vi "ELVIS III v1.0 RPC Get Session.vi"(8 "error in (no error)":errorcluster) -> (0 "error out":errorcluster, 3 "Session":u32)   [LabVIEW 2021]
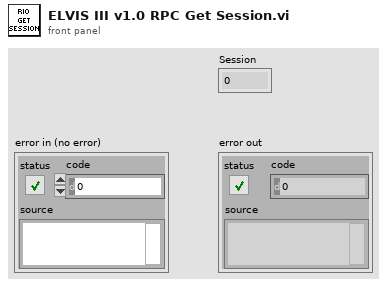
[diagram p1: front panel]
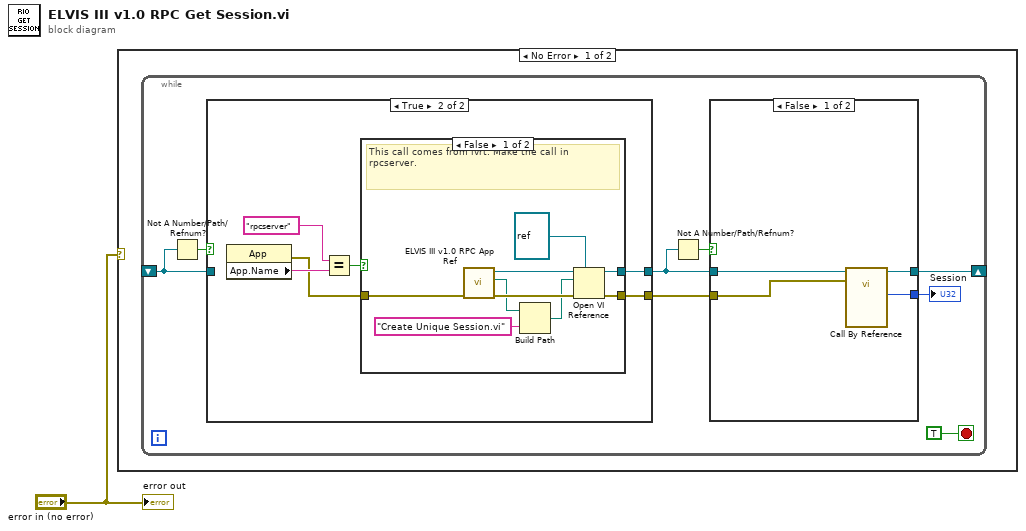
[diagram p0: block diagram]
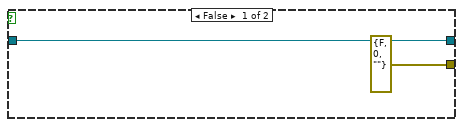
[diagram p2: hidden frame]
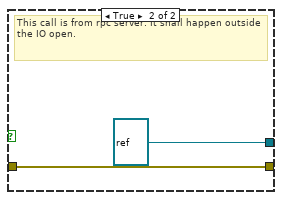
[diagram p3: hidden frame]
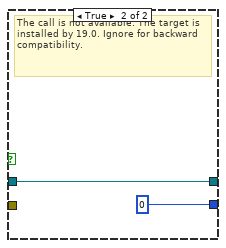
[diagram p4: hidden frame]
diagram:
  n1 = case shown="No Error" "error in (no error)" {
    frame No Error {
      n2 = while {
        shift-right: [w6] -> _
        shift-left: _ -> [w4]
        stop <- TRUE stop-if-true
        n3 = Not A Number/Path/Refnum?(number/path/refnum=w4) -> (NaN/Path/Refnum?=w5:bool)
        n4 = case shown="True" w5 {
          tunnel: [w11 w14] -> w8
          tunnel: w4 -> [w11 _]
          tunnel: [errorcluster {"status"=FALSE, "code"=0, "source"=""} ("error out") w12] -> w3
          frame False {
          }
          frame True {
            n5 = property class="App"() -> (error out=w13:errorcluster, "App.Name"=w17:string)  [unwired: 2 in, 1 out]
            n6 = Equal?(x="rpcserver" ("Application:Name"), y=w17) -> (x = y?=w16:bool)
            n7 = case shown="False" w16 {
              tunnel: [w24 refnum<vi> refnum ("type specifier VI Refnum (for type only)")] -> w14
              tunnel: w13 -> [w22 w27]
              tunnel: [w23 w27] -> w12
              frame False {
                # "This call comes from lvrt. Make the call in rpcserver."
                n8 = call <vilib>:"ELVIS III v1.0 RPC App Ref.vi"() -> ("Lib Path"=w21:path, "RPC Reference"=w19:refnum<vi>)  [unwired: 10 in]
                n9 = Build Path(base path=w21, name or relative path="Create Unique Session.vi") -> (appended path=w18:path)
                n10 = Open VI Reference(type specifier VI Refnum (for type only)=refnum<vi> refnum, application reference (local)=w19, vi path=w18, error in (no error)=w22) -> (vi reference=w24:refnum<vi>, error out=w23:errorcluster)  [unwired: 2 in]
              }
              frame True {
                # "This call is from rpc server. It shall happen outside the IO open."
              }
            }
          }
        }
        n11 = Not A Number/Path/Refnum?(number/path/refnum=w8) -> (NaN/Path/Refnum?=w9:bool)
        n12 = case shown="False" w9 {
          tunnel: w8 -> [w31 w33]
          tunnel: [w30 w33] -> w6
          tunnel: w3 -> [w29 _]
          tunnel: [w28 u32 0 ("Session")] -> w2
          frame False {
            n13 = call-by-ref "?"(reference=w31, error in=w29) -> (reference out=w30:refnum<vi>, "Session"=w28:u32)  [unwired: 11 in, 1 out]
          }
          frame True {
            # "The call is not available. The target is installed by 19.0. Ignore for backward compatibility."
          }
        }
        "Session" <- w2
      }
    }
    frame Error {
    }
  }
  "error out" <- "error in (no error)"
